vi "optogeneticsTarget3DMultiple.vi"(0 "X (camera space)":i32[](array[numeric]), 1 "Y (camera space)":i32[](array[numeric]), 2 "Z (imaging space)":i32[](array[numeric]), 3 "piezoEtlPositions":dbl[](array[numeric]), 5 "fire (true: needed for multi-neuron)":bool=TRUE, 6 "stimulationTime (s)":dbl=1.0, 7 "pharosNTrains":i32, 8 "pharosRepRateDivider":u32=1, 9 "pharosTimeBtwTrains (s)":dbl, 10 "repeats":i32=1, 12 "intervalBtwnStimulations (s)":dbl=1.0) -> ()   [LabVIEW 2017]
uses:
  globalUtilities.vi
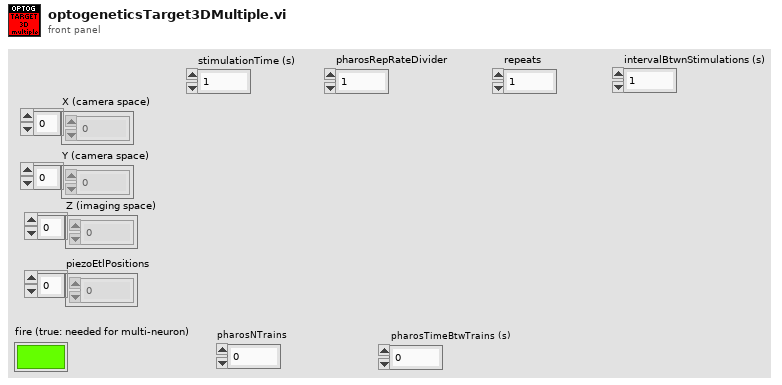
[diagram p1: front panel]
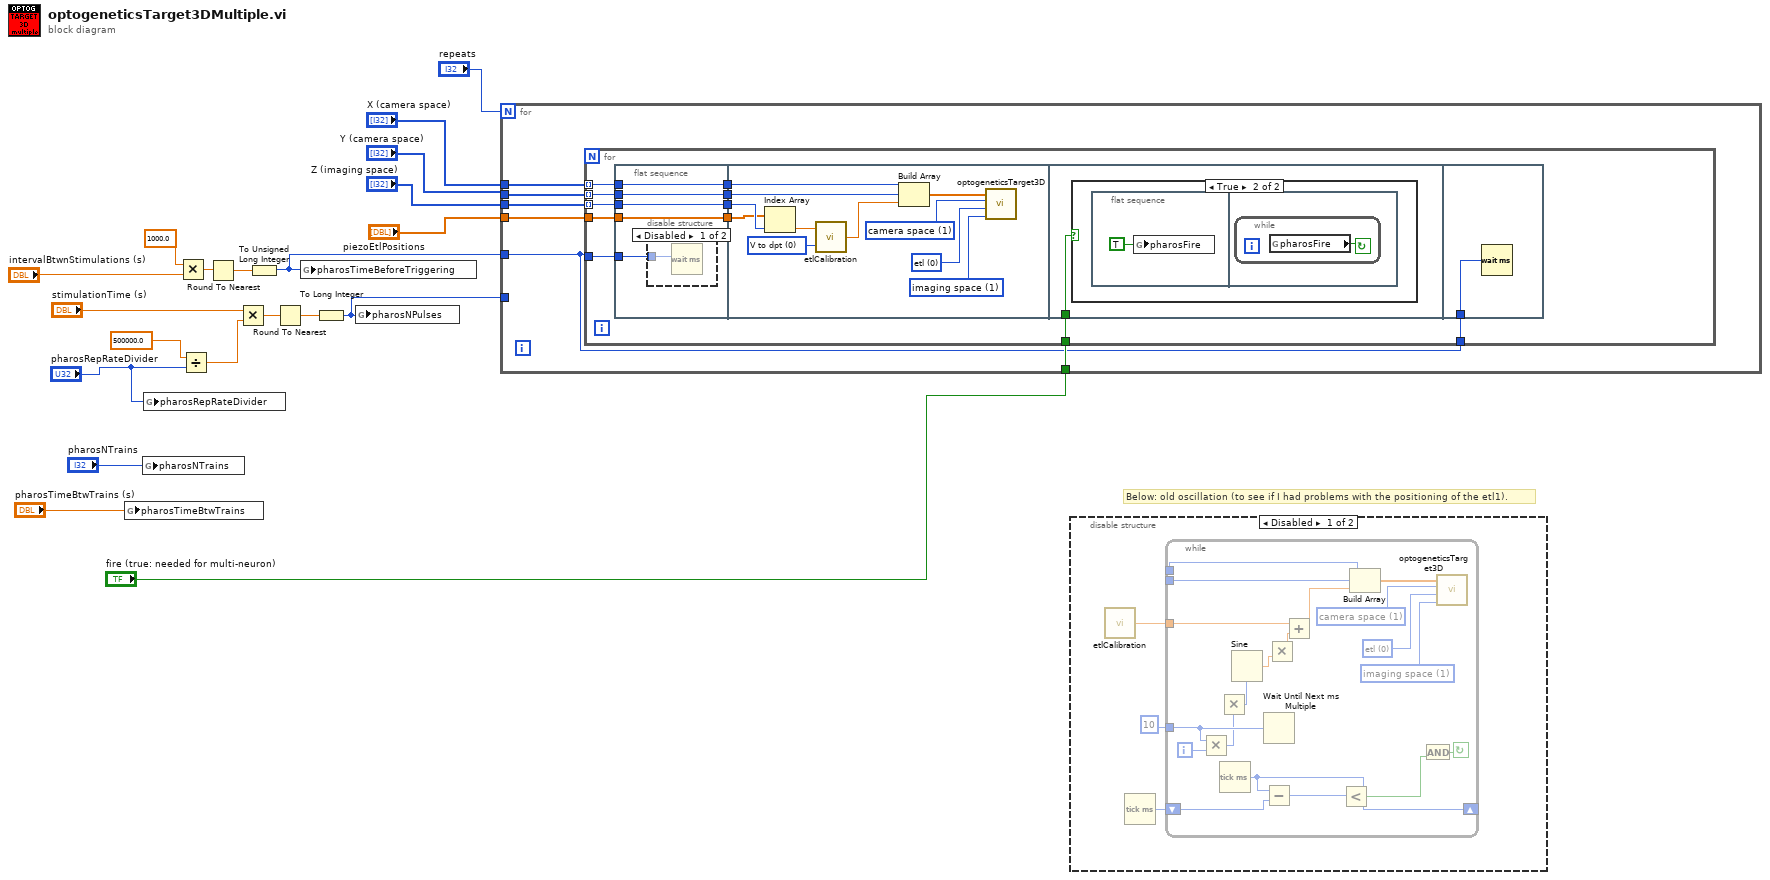
[diagram p0: block diagram]
diagram:
  # "Below: old oscillation (to see if I had problems with the positioning of the etl1)."
  n1 = global write "globalUtilities.vi" "pharosTimeBtwTrains"("pharosTimeBtwTrains (s)") -> ()
  n2 = global write "globalUtilities.vi" "pharosNTrains"("pharosNTrains") -> ()
  n3 = global write "globalUtilities.vi" "pharosRepRateDivider"("pharosRepRateDivider") -> ()
  n4 = Multiply(x=1000.0, y="intervalBtwnStimulations (s)") -> (x*y=w5:dbl)
  n5 = Divide(x=500000.0 ("y"), y="pharosRepRateDivider") -> (x/y=w13:dbl)
  n6 = Round To Nearest(number=w5) -> (nearest integer value=w6:dbl)
  n7 = Multiply(x="stimulationTime (s)", y=w13) -> (x*y=w12:dbl)
  n8 = To Unsigned Long Integer(number=w6) -> (unsigned 32bit integer=w4:u32)
  n9 = Round To Nearest(number=w12) -> (nearest integer value=w11:dbl)
  n10 = global write "globalUtilities.vi" "pharosTimeBeforeTriggering"(w4) -> ()
  n11 = To Long Integer(number=w11) -> (32bit integer=w9:i32)
  n12 = global write "globalUtilities.vi" "pharosNPulses"(w9) -> ()
  n13 = for {
    N: "repeats" -> [_]
    tunnel: "X (camera space)" -> [w26]
    tunnel: "Y (camera space)" -> [w25]
    tunnel: "Z (imaging space)" -> [w24]
    tunnel: "piezoEtlPositions" -> [w23]
    tunnel: w9 -> [_]
    tunnel: w4 -> [w21]
    tunnel: "fire (true: needed for multi-neuron)" -> [w22]
    n14 = for {
      tunnel: w26 -> [w37] mode=indexing
      tunnel: w25 -> [w36] mode=indexing
      tunnel: w24 -> [w35] mode=indexing
      tunnel: w23 -> [w34]
      tunnel: w21 -> [w29]
      tunnel: w22 -> [w28]
      tunnel: w21 -> [w27]
      n15 = flat-sequence {
        tunnel: w34 -> [w39]
        tunnel: w35 -> [w40]
        tunnel: w36 -> [w41]
        tunnel: w37 -> [w42]
        tunnel: [w42] -> w33
        tunnel: [w41] -> w32
        tunnel: [w40] -> w31
        tunnel: [w39] -> w30
        tunnel: w29 -> [w38]
        tunnel: w33 -> [w54]
        tunnel: w32 -> [w53]
        tunnel: w31 -> [w52]
        tunnel: w30 -> [w48]
        tunnel: w28 -> [w55]
        tunnel: w27 -> [w58]
        frame #0 {
          n16 = disable-structure shown="Disabled" {
            disable-tunnel: w38 -> [w43 _]
            frame Disabled {
              n17 = Wait (ms)(milliseconds to wait=w43) -> ()  [unwired: 1 out]
            }
            frame Enabled {
            }
          }
        }
        frame #1 {
          w44 = u16 1 items=["optogenetics space", "imaging space"] ("z mode")
          w45 = u16 0 items=["etl", "piezo"] ("z device")
          w46 = u16 1 items=["galvo space", "camera space"] ("xy mode")
          w50 = u16 0 items=["V to dpt", "dpt to V"] ("mode")
          n18 = Index Array(array=w48, index=w52) -> (element=w51:dbl)
          n19 = call "etlCalibration.vi"("mode"=w50, "in"=w51) -> ("out"=w49:dbl)
          n20 = Build Array(w54, w53, w49) -> (w47:dbl[])
          n21 = call "optogeneticsTarget3D.vi"("z mode"=w44, "z device"=w45, "xy mode"=w46, "xyz"=w47) -> ()  [unwired: 1 in]
        }
        frame #2 {
          n22 = case shown="True" w55 {
            frame False {
            }
            frame True {
              n23 = flat-sequence {
                frame #0 {
                  n24 = global write "globalUtilities.vi" "pharosFire"(TRUE ("pharosFire")) -> ()
                }
                frame #1 {
                  n25 = while {
                    stop <- w57 continue-if-true
                    n26 = global read "globalUtilities.vi" "pharosFire"() -> (w57:bool)
                  }
                }
              }
            }
          }
        }
        frame #3 {
          n27 = Wait (ms)(milliseconds to wait=w58) -> ()  [unwired: 1 out]
        }
      }
    }
  }
  n28 = disable-structure shown="Disabled" {
    frame Disabled {
      n29 = call "etlCalibration.vi"() -> ("out"=w59:dbl)  [unwired: 2 in]
      n30 = Tick Count (ms)() -> (millisecond timer value=w61:u32)
      n31 = while {
        tunnel: _ -> [w82]
        tunnel: _ -> [w81]
        tunnel: w59 -> [w76]
        tunnel: u32 10 ("millisecond multiple") -> [w70]
        shift-right: [w66] -> _
        shift-left: w61 -> [w67]
        i -> [w71]
        stop <- w62 continue-if-true
        w77 = u16 1 items=["optogenetics space", "imaging space"] ("z mode")
        w78 = u16 0 items=["etl", "piezo"] ("z device")
        w79 = u16 1 items=["galvo space", "camera space"] ("xy mode")
        n32 = Multiply(x=w70, y=w71) -> (x*y=w69:u32)
        n33 = Multiply(y=w69) -> (x*y=w68:u32)  [unwired: 1 in]
        n34 = Tick Count (ms)() -> (millisecond timer value=w66:u32)
        n35 = Sine(x=w68) -> (sin(x)=w72:dbl)
        n36 = Wait Until Next ms Multiple(millisecond multiple=w70) -> ()  [unwired: 1 out]
        n37 = Subtract(x=w66, y=w67) -> (x-y=w65:u32)
        n38 = Multiply(y=w72) -> (x=w73:dbl, x*y=w74:dbl)
        n39 = Add(x=w76, y=w74) -> (x+y=w75:dbl)
        n40 = Less?(x=w65) -> (y=w64:u32, x < y?=w63:bool)
        n41 = Build Array(w82, w81, w75) -> (w80:dbl[])
        n42 = And(y=w63) -> (x .and. y?=w62:bool)  [unwired: 1 in]
        n43 = call "optogeneticsTarget3D.vi"("z mode"=w77, "z device"=w78, "xy mode"=w79, "xyz"=w80) -> ()  [unwired: 1 in]
      }
    }
    frame Enabled {
    }
  }
